vi "Gitlab OAuth Test.vi"() -> ()   [LabVIEW 2020]
uses:
  OauthClient/OAuthClient.lvclass
  Oauth2/Oauth2.lvclass/Oauth2.ctl
  Oauth2.GitLab/Oauth2.GitLab.lvclass
  C:/Data/1_Projects/CIGH_Oauth2/source/Oauth2/Oauth2.lvclass
  Oauth2/Oauth2.lvclass
  <vilib>/LabVIEW Open Source Project/OpenURI/uri/URI.lvclass
  <vilib>/httpClient/LabVIEWHTTPClient.lvlib
panel:
  out "REST API Error":errorcluster
  in  "Query API Version":bool
  in  "Refresh":bool
  in  "Authorize":bool
  out "Gitlab Version":string
  out "HTTP Response Headers":string
  out "Redirect URI":string
  out "granted scopes":string[](array[string])
  out "Created At":u32
  out "Expires In":u32
  out "Refresh Token":string
  in  "GitLab Client Secret":string
  in  "GitLab Client ID":string
  out "GitLab Access Token":string
  out "Oauth Error":errorcluster
  in  "GitLab Authorization Server URI":string="https://gitlab.com"
  # "Gitlab Application API Access Example"
  # "G Open Source Project for LabVIEW\nhttps://github.com/LabVIEW-Open-Source/Oauth2"
  # "1- Get a Client ID and Client Secret from the application's admin. \n\n          * To access your own server, log into your site, create an application and set the access scope.\n             you want. \n          * This Oauth2.0 API uses the following redirect URL: http://localhost:58888/Oauth2/Redirect\n          * Record the client ID and client secret and fill in the fields below."
  # "2- Set the Gitlab Authorization server address, without the relative \"oauth/authorize\" path.\n         * If using Gitlab's cloud, the URI is \"https://gitlab.com\"\n         * With your own domain, it could be \"https://gitlab.example.com\" or something similar."
  # "0: Never expired"
  # "3- Get an Access Token. You will be redirected your Gitlab's Authorization Server URI\n              * Use the \"Get Access Token\" button on the top right of this page.\n\n4- Once you have authenticated yourself, you will receive an access token.\n              * Use the \"Refresh Token\" button to request a fresh token\n                       OR\n              * Use the Access Token to query the Gitlab API (example is to retrieve the Gitlab Version)"
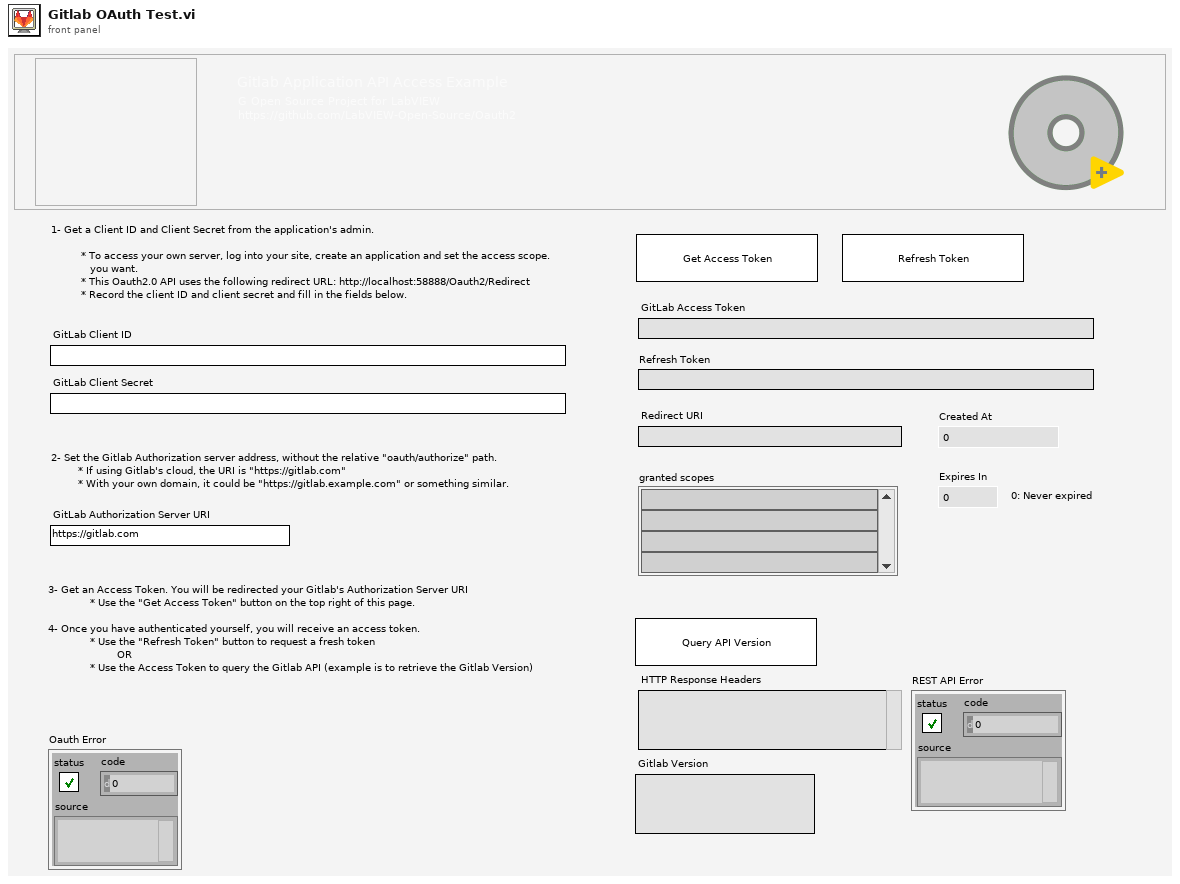
[diagram p1: front panel]
types:
  T1 = enum8{"Enabled", "Disabled", "Disabled and Grayed Out"}
  T2 = cluster{"Oauth2":refnum<class "Oauth2.GitLab.lvclass">, "GitLab Authorization Server URI":string}
  T3 = typedef "LabVIEWHTTPClient.lvlib/ClientHandle.ctl" = refnum<k1>
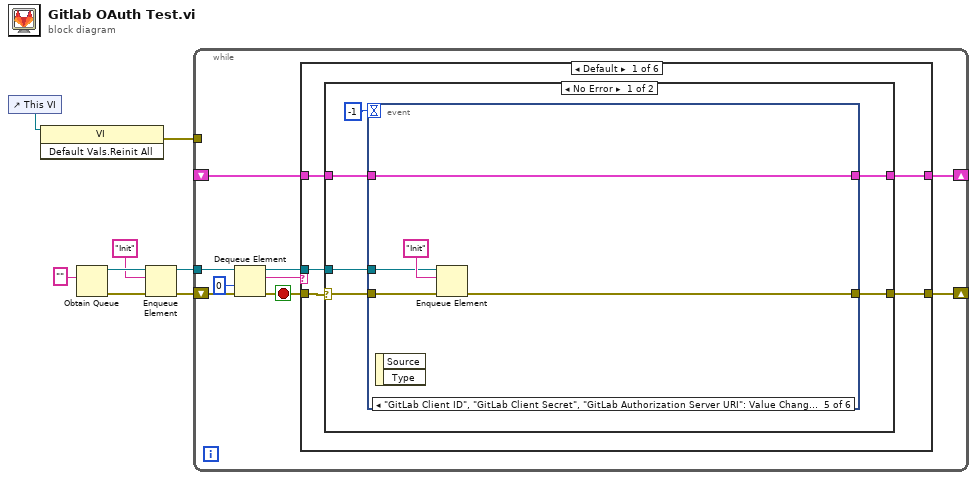
[diagram p0: block diagram]
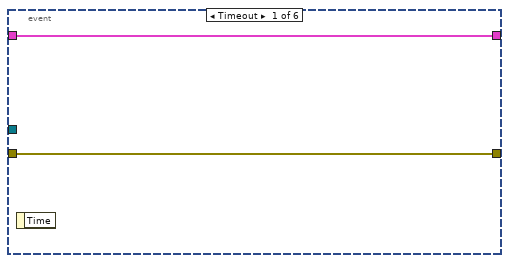
[diagram p2: hidden frame]
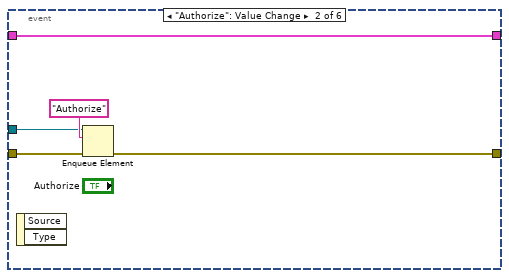
[diagram p3: hidden frame]
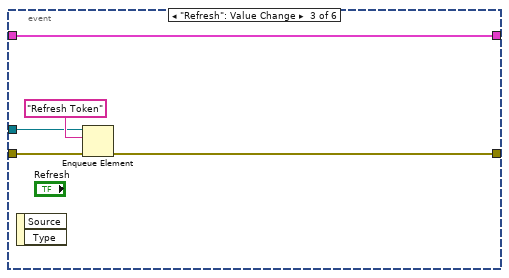
[diagram p4: hidden frame]
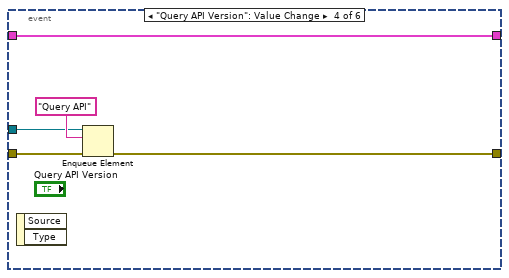
[diagram p5: hidden frame]
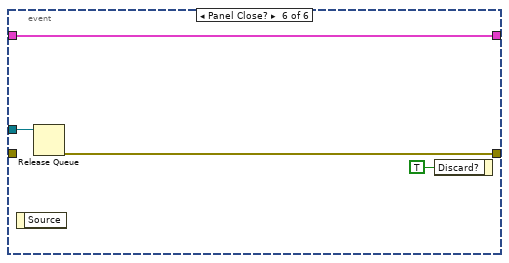
[diagram p6: hidden frame]
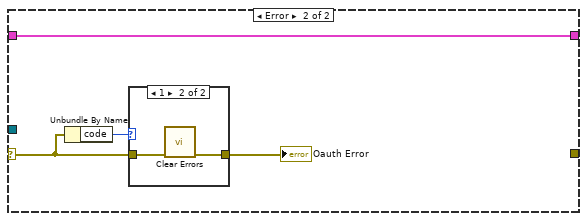
[diagram p7: hidden frame]
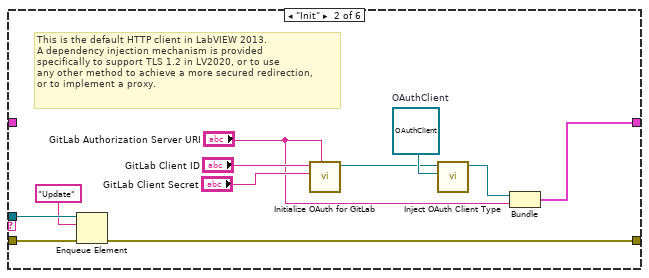
[diagram p9: hidden frame]
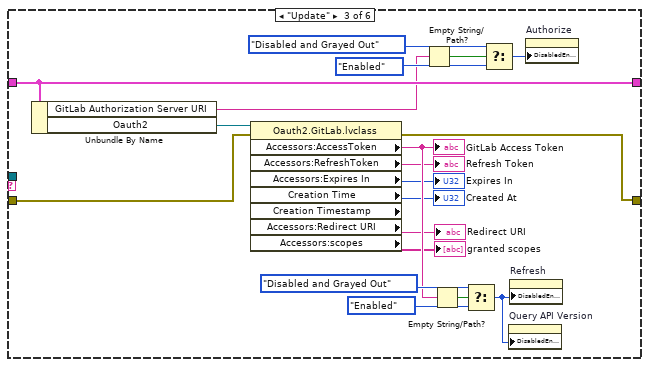
[diagram p10: hidden frame]
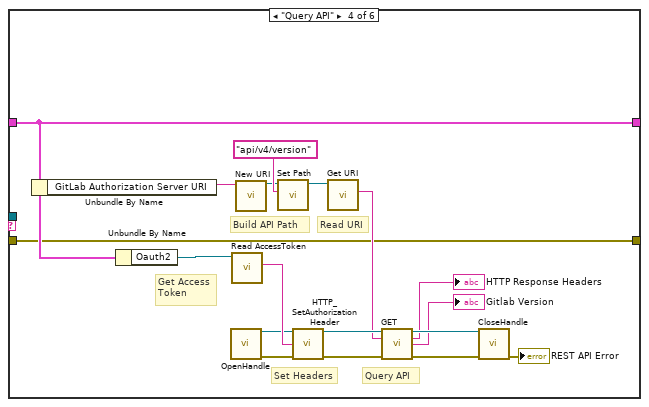
[diagram p11: hidden frame]
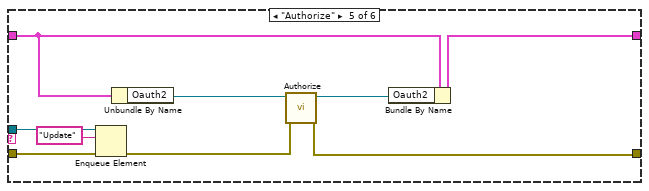
[diagram p12: hidden frame]
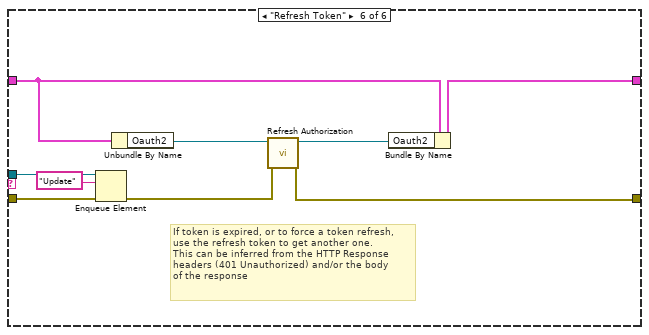
[diagram p13: hidden frame]
diagram:
  n1 = control-ref of="This VI"() -> (w2:refnum<vi>)
  n2 = invoke class="VI" method="Default Vals.Reinit All"(reference=w2) -> (error out=w1:errorcluster)  [unwired: 2 in, 2 out]
  n3 = Obtain Queue(element data type="") -> (queue out=w5:refnum<queue>, error out=w7:errorcluster)  [unwired: 4 in, 1 out]
  n4 = Enqueue Element(queue=w5, element="Init", error in (no error)=w7) -> (queue out=w4:refnum<queue>, error out=w6:errorcluster)  [unwired: 1 in, 1 out]
  n5 = while {
    tunnel: w4 -> [w17]
    shift-right: [w12] -> _
    shift-left: _ -> [w11]
    shift-right: [w9] -> _
    shift-left: w6 -> [w13]
    tunnel: w1 -> [_]
    stop <- w10 stop-if-true
    n6 = Dequeue Element(queue=w17, timeout in ms (-1)=0, error in (no error)=w13) -> (queue out=w14:refnum<queue>, element=w15:string, error out=w10:errorcluster)  [unwired: 1 out]
    n7 = case shown="Default" w15 {
      tunnel: w14 -> [w22 w71 _ _ w112 w124]
      tunnel: [w21 w72 w91 w106 w114 w126] -> w12
      tunnel: w11 -> [w20 _ w91 w106 w115 w127]
      tunnel: w10 -> [w19 w68 w81 w94 w111 w123]
      tunnel: [w18 w69 w80 w94 w117 w119] -> w9
      frame Default {
        n8 = case shown="No Error" w19 {
          selector: w19 -> [w23 w57]
          tunnel: w22 -> [w27 _]
          tunnel: [w26 w58] -> w21
          tunnel: w20 -> [w25 w58]
          tunnel: [w24 _] -> w18
          frame No Error {
            n9 = event shown="[4] \"GitLab Client ID\", \"GitLab Client Secret\", \"GitLab Authorization Server URI\": Value Change" {
              selector: _ -> [_ _ _ _ _ _]
              dyn-events: _ -> [_ _ _ _ _ _]
              timeout: -1 -> [_ _ _ _ _ _]
              tunnel: w27 -> [_ w34 w39 w44 w49 w54]
              tunnel: [w30 w32 w37 w42 w47 w52] -> w26
              tunnel: w25 -> [w30 w32 w37 w42 w47 w52]
              tunnel: [w29 w31 w36 w41 w46 w51] -> w24
              tunnel: w23 -> [w29 w33 w38 w43 w48 _]
              event Timeout {
                n10 = event-data() -> ()  [unwired: 1 in, 1 out]
              }
              event "Authorize": Value Change {
                n11 = event-data() -> ()  [unwired: 1 in, 2 out]
                n12 = Enqueue Element(queue=w34, element="Authorize", error in (no error)=w33) -> (error out=w31:errorcluster)  [unwired: 1 in, 2 out]
              }
              event "Refresh": Value Change {
                n13 = event-data() -> ()  [unwired: 1 in, 2 out]
                n14 = Enqueue Element(queue=w39, element="Refresh Token", error in (no error)=w38) -> (error out=w36:errorcluster)  [unwired: 1 in, 2 out]
              }
              event "Query API Version": Value Change {
                n15 = event-data() -> ()  [unwired: 1 in, 2 out]
                n16 = Enqueue Element(queue=w44, element="Query API", error in (no error)=w43) -> (error out=w41:errorcluster)  [unwired: 1 in, 2 out]
              }
              event "GitLab Client ID", "GitLab Client Secret", "GitLab Authorization Server URI": Value Change {
                n17 = event-data() -> ()  [unwired: 1 in, 2 out]
                n18 = Enqueue Element(queue=w49, element="Init", error in (no error)=w48) -> (error out=w46:errorcluster)  [unwired: 1 in, 2 out]
              }
              event Panel Close? {
                n19 = event-data() -> ()  [unwired: 1 in, 1 out]
                n20 = Release Queue(queue=w54) -> (error out=w51:errorcluster)  [unwired: 2 in, 2 out]
                n21 = event-data("Discard?"=TRUE) -> ()  [unwired: 1 in, 1 out]
              }
            }
          }
          frame Error {
            n22 = Unbundle By Name(w57) -> ("code"=w55:i32)
            n23 = case shown="1" w55 {
              tunnel: w57 -> [w59 w61]
              tunnel: [w59 w60] -> w56
              frame Default {
              }
              frame 1 {
                n24 = call <vilib>:"Clear Errors.vi"("error in (no error)"=w61) -> ("error out"=w60:errorcluster)  [unwired: 5 in, 1 out]
              }
            }
            "Oauth Error" <- w56
          }
        }
      }
      frame "Init" {
        w65 = refnum<class "OAuthClient.lvclass"> refnum  # OAuthClient
        # "This is the default HTTP client in LabVIEW 2013.\nA dependency injection mechanism is provided\nspecifically to support TLS 1.2 in LV2020, or to use\nany other method to achieve a more secured redirection, \nor to implement a proxy."
        n25 = Enqueue Element(queue=w71, element="Update", error in (no error)=w68) -> (error out=w69:errorcluster)  [unwired: 1 in, 2 out]
        n26 = call "Initialize OAuth for GitLab.vi"("Authorization Server URI"="GitLab Authorization Server URI", "Client Secret"="GitLab Client Secret", "Client ID"="GitLab Client ID") -> ("Oauth2.GitLab"=w64:refnum<class "Oauth2.GitLab.lvclass">)  [unwired: 7 in, 1 out]
        n27 = call "Inject OAuth Client Type.vi"("OAuthClient"=w65, "Oauth2 in"=w64) -> ("Oauth2"=w63:refnum<class "Oauth2.GitLab.lvclass">)  [unwired: 9 in]
        n28 = Bundle("Oauth2"=w63, "GitLab Authorization Server URI"="GitLab Authorization Server URI") -> (w72:T2)  [unwired: 1 in]
      }
      frame "Update" {
        n29 = Unbundle By Name(w91) -> ("GitLab Authorization Server URI"=w85:string, "Oauth2"=w86:refnum<class "Oauth2.GitLab.lvclass">)
        n30 = property class="Oauth2.GitLab.lvclass" props=["Accessors:AccessToken", "Accessors:RefreshToken", "Accessors:Expires In", "Creation Time", "Creation Timestamp", "Accessors:Redirect URI", "Accessors:scopes"](reference=w86, error in=w81) -> (error out=w80:errorcluster, "Accessors:AccessToken"=w79:string, "Accessors:RefreshToken"=→"Refresh Token":string, "Accessors:Expires In"=→"Expires In":u32, "Creation Time"=→"Created At":u32, "Accessors:Redirect URI"=→"Redirect URI":string, "Accessors:scopes"=→"granted scopes":string[])  [unwired: 2 out]
        "GitLab Access Token" <- w79
        n31 = Empty String/Path?(string/path=w85) -> (empty?=w88:bool)
        n32 = Empty String/Path?(string/path=w79) -> (empty?=w84:bool)
        n33 = Select(t=T1."Disabled and Grayed Out" ("Disabled"), s=w84, f=T1."Enabled" ("Disabled")) -> (s? t:f=w73:T1)
        n34 = Select(t=T1."Disabled and Grayed Out" ("Disabled"), s=w88, f=T1."Enabled" ("Disabled")) -> (s? t:f=w87:T1)
        n35 = property on="Query API Version" class="Bool"("DisabledEnum"=w73) -> ()  [unwired: 2 in, 2 out]
        n36 = property on="Refresh" class="Bool"("DisabledEnum"=w73) -> ()  [unwired: 2 in, 2 out]
        n37 = property on="Authorize" class="Bool"("DisabledEnum"=w87) -> ()  [unwired: 2 in, 2 out]
      }
      frame "Query API" {
        # "Query API"
        # "Set Headers"
        # "Get Access\nToken"
        # "Read URI"
        # "Build API Path"
        n38 = Unbundle By Name(w106) -> ("GitLab Authorization Server URI"=w102:string)
        n39 = Unbundle By Name(w106) -> ("Oauth2"=w107:refnum<class "Oauth2.GitLab.lvclass">)
        n40 = call <vilib>:"OpenHandle.vi"() -> ("client handle out"=w108:T3, "error out"=w99:errorcluster)  [unwired: 14 in]
        n41 = call "Read AccessToken.vi"("Oauth2 in"=w107) -> ("Access Token"=w109:string)  [unwired: 8 in, 2 out]
        n42 = call <vilib>:"New URI.vi"("URI"=w102) -> ("URI"=w103:refnum<class "URI.lvclass">)  [unwired: 9 in, 1 out]
        n43 = call <vilib>:"Set Path.vi"("path"="api/v4/version", "URI in"=w103) -> ("URI out"=w105:refnum<class "URI.lvclass">)  [unwired: 8 in, 1 out]
        n44 = call "HTTP_SetAuthorizationHeader.vi"("Client Handle"=w108, "Access Token"=w109, "error in (no error)"=w99) -> ("client handle dup"=w101:T3, "error out"=w98:errorcluster)  [unwired: 11 in]
        n45 = call <vilib>:"Get URI.vi"("URI in"=w105) -> ("URI String"=w100:string)  [unwired: 8 in, 2 out]
        n46 = call <vilib>:"GET.vi"("client handle"=w101, "url"=w100, "error in (no error)"=w98) -> ("client handle out"=w97:T3, "headers"=→"HTTP Response Headers":string, "body"=→"Gitlab Version":string, "error out"=w96:errorcluster)  [unwired: 9 in]
        n47 = call <vilib>:"CloseHandle.vi"("client handle"=w97, "error in (no error)"=w96) -> ("error out"=→"REST API Error":errorcluster)  [unwired: 13 in]
      }
      frame "Authorize" {
        n48 = Enqueue Element(queue=w112, element="Update", error in (no error)=w111) -> (error out=w110:errorcluster)  [unwired: 1 in, 2 out]
        n49 = Unbundle By Name(w115) -> ("Oauth2"=w118:refnum<class "Oauth2.GitLab.lvclass">)
        n50 = call "Authorize.vi"("error in (no error)"=w110, "Oauth2 in"=w118) -> ("error out"=w117:errorcluster, "Oauth2 out"=w116:refnum<class "Oauth2.GitLab.lvclass">)  [unwired: 7 in, 1 out]
        n51 = Bundle By Name(cluster=w115, "Oauth2"=w116) -> (w114:T2)
      }
      frame "Refresh Token" {
        # "If token is expired, or to force a token refresh, \nuse the refresh token to get another one.\nThis can be inferred from the HTTP Response\nheaders (401 Unauthorized) and/or the body\nof the response"
        n52 = Enqueue Element(queue=w124, element="Update", error in (no error)=w123) -> (error out=w120:errorcluster)  [unwired: 1 in, 2 out]
        n53 = Unbundle By Name(w127) -> ("Oauth2"=w122:refnum<class "Oauth2.GitLab.lvclass">)
        n54 = call "Refresh Authorization.vi"("error in (no error)"=w120, "Oauth2 in"=w122) -> ("error out"=w119:errorcluster, "Oauth2 out"=w121:refnum<class "Oauth2.GitLab.lvclass">)  [unwired: 7 in, 1 out]
        n55 = Bundle By Name(cluster=w127, "Oauth2"=w121) -> (w126:T2)
      }
    }
  }
